vi "Main.vi"(7 "sweep rate, /min":dbl=0.2, 8 "sweep to:":dbl=-0.5, 9 "sweep":T6(radio)=enum."time_sweep") -> ()   [LabVIEW 2017] (continued)
                n3333 = property on="Figure_axis" class="Arr (strict)"("Value"=w4305) -> ()  [unwired: 2 in, 2 out]
                n3334 = property on="data_caption" class="Str"("Value"=w4307) -> ()  [unwired: 2 in, 2 out]
              }
              frame #32 {
                # "2182A 4 channel 1 measure (2182A_4_ch1)"
                n3335 = local read "2182A 4 ch1"() -> (w4324:bool)
                n3336 = property on="Figure_axis" class="Arr (strict)"() -> ("Value"=w4321:string[])  [unwired: 2 in, 2 out]
                n3337 = property on="data_caption" class="Str"() -> ("Value"=w4323:string)  [unwired: 2 in, 2 out]
                n3338 = case shown="True" w4324 {
                  tunnel: w4323 -> [w4326 w4332]
                  tunnel: [w4326 w4331] -> w4322
                  tunnel: w4321 -> [w4325 w4329]
                  tunnel: [w4325 w4327] -> w4320
                  frame False {
                    # "not measure 2182A 4 channel 1 (2182A_4_ch1)"
                  }
                  frame True {
                    w4328 = "2182A_4_ch1"
                    # "measure 2182A 4 channel 1 (2182A_4_ch1)"
                    n3339 = local read "2182A 4 addr"() -> (w4333:u8)
                    n3340 = Number To Decimal String(number=w4333) -> (decimal integer string=w4334:string)  [unwired: 1 in]
                    n3341 = GPIB Clear(3:w4334) -> ()  [unwired: 1 in, 2 out]
                    n3342 = Build Array (concatenate)(w4329, w4328) -> (w4327:string[])
                    n3343 = Concatenate Strings(w4332, w4328, "\t") -> (w4331:string)
                  }
                }
                n3344 = property on="Figure_axis" class="Arr (strict)"("Value"=w4320) -> ()  [unwired: 2 in, 2 out]
                n3345 = property on="data_caption" class="Str"("Value"=w4322) -> ()  [unwired: 2 in, 2 out]
              }
              frame #33 {
                # "2182A 4 channel 2 measure (2182A_4_ch2)"
                n3346 = local read "2182A 4 ch2"() -> (w4339:bool)
                n3347 = property on="Figure_axis" class="Arr (strict)"() -> ("Value"=w4336:string[])  [unwired: 2 in, 2 out]
                n3348 = property on="data_caption" class="Str"() -> ("Value"=w4338:string)  [unwired: 2 in, 2 out]
                n3349 = case shown="True" w4339 {
                  tunnel: w4338 -> [w4341 w4347]
                  tunnel: [w4341 w4346] -> w4337
                  tunnel: w4336 -> [w4340 w4344]
                  tunnel: [w4340 w4342] -> w4335
                  frame False {
                    # "not measure 2182A 4 channel 2 (2182A_4_ch2)"
                  }
                  frame True {
                    w4343 = "2182A_4_ch2"
                    # "measure 2182A 4 channel 2 (2182A_4_ch2)"
                    n3350 = local read "2182A 4 addr"() -> (w4348:u8)
                    n3351 = Number To Decimal String(number=w4348) -> (decimal integer string=w4349:string)  [unwired: 1 in]
                    n3352 = GPIB Clear(3:w4349) -> ()  [unwired: 1 in, 2 out]
                    n3353 = Build Array (concatenate)(w4344, w4343) -> (w4342:string[])
                    n3354 = Concatenate Strings(w4347, w4343, "\t") -> (w4346:string)
                  }
                }
                n3355 = property on="Figure_axis" class="Arr (strict)"("Value"=w4335) -> ()  [unwired: 2 in, 2 out]
                n3356 = property on="data_caption" class="Str"("Value"=w4337) -> ()  [unwired: 2 in, 2 out]
              }
              frame #34 {
                # "2636A smua measure voltage (2636A_smua_v)"
                n3357 = local read "2636A smua meas v"() -> (w4354:bool)
                n3358 = property on="Figure_axis" class="Arr (strict)"() -> ("Value"=w4351:string[])  [unwired: 2 in, 2 out]
                n3359 = property on="data_caption" class="Str"() -> ("Value"=w4353:string)  [unwired: 2 in, 2 out]
                n3360 = case shown="True" w4354 {
                  tunnel: w4353 -> [w4356 w4367]
                  tunnel: [w4356 w4366] -> w4352
                  tunnel: w4351 -> [w4355 w4364]
                  tunnel: [w4355 w4362] -> w4350
                  frame False {
                    # "not measure voltage on 2636A smua (2636A_smua_v)"
                  }
                  frame True {
                    w4363 = "2636A_smua_v"
                    # "measure voltage on 2636A smua (2636A_smua_v)"
                    n3361 = local read "2336A addr"() -> (w4358:refnum<visa-resource-name>)
                    n3362 = VISA Open(VISA resource name=w4358) -> (VISA resource name=w4357:refnum<visa-resource-name>, error out=w4359:errorcluster)  [unwired: 4 in]
                    n3363 = VISA Clear(VISA resource name=w4357, error in (no error)=w4359) -> (VISA resource name out=w4361:refnum<visa-resource-name>)  [unwired: 1 out]
                    n3364 = property class="Instr"(reference=w4361, "General Settings:Timeout Value"=u32 10000) -> ()  [unwired: 1 in, 2 out]
                    n3365 = Build Array (concatenate)(w4364, w4363) -> (w4362:string[])
                    n3366 = Concatenate Strings(w4367, w4363, "\t") -> (w4366:string)
                  }
                }
                n3367 = property on="Figure_axis" class="Arr (strict)"("Value"=w4350) -> ()  [unwired: 2 in, 2 out]
                n3368 = property on="data_caption" class="Str"("Value"=w4352) -> ()  [unwired: 2 in, 2 out]
              }
              frame #35 {
                # "2636A smua measure current (2636A_smua_i)"
                n3369 = local read "2636A smua meas i"() -> (w4372:bool)
                n3370 = property on="Figure_axis" class="Arr (strict)"() -> ("Value"=w4369:string[])  [unwired: 2 in, 2 out]
                n3371 = property on="data_caption" class="Str"() -> ("Value"=w4371:string)  [unwired: 2 in, 2 out]
                n3372 = case shown="True" w4372 {
                  tunnel: w4371 -> [w4374 w4385]
                  tunnel: [w4374 w4384] -> w4370
                  tunnel: w4369 -> [w4373 w4382]
                  tunnel: [w4373 w4380] -> w4368
                  frame False {
                    # "not measure current on 2636A smua (2636A_smua_i)"
                  }
                  frame True {
                    w4381 = "2636A_smua_i"
                    # "measure current on 2636A smua (2636A_smua_i)"
                    n3373 = local read "2336A addr"() -> (w4377:refnum<visa-resource-name>)
                    n3374 = VISA Open(VISA resource name=w4377) -> (VISA resource name=w4376:refnum<visa-resource-name>, error out=w4375:errorcluster)  [unwired: 4 in]
                    n3375 = VISA Clear(VISA resource name=w4376, error in (no error)=w4375) -> (VISA resource name out=w4378:refnum<visa-resource-name>)  [unwired: 1 out]
                    n3376 = Build Array (concatenate)(w4382, w4381) -> (w4380:string[])
                    n3377 = property class="Instr"(reference=w4378, "General Settings:Timeout Value"=u32 10000) -> ()  [unwired: 1 in, 2 out]
                    n3378 = Concatenate Strings(w4385, w4381, "\t") -> (w4384:string)
                  }
                }
                n3379 = property on="Figure_axis" class="Arr (strict)"("Value"=w4368) -> ()  [unwired: 2 in, 2 out]
                n3380 = property on="data_caption" class="Str"("Value"=w4370) -> ()  [unwired: 2 in, 2 out]
              }
              frame #36 {
                # "2636A smub measure voltage (2636A_smub_v)"
                n3381 = local read "2636A smub meas v"() -> (w4390:bool)
                n3382 = property on="Figure_axis" class="Arr (strict)"() -> ("Value"=w4387:string[])  [unwired: 2 in, 2 out]
                n3383 = property on="data_caption" class="Str"() -> ("Value"=w4389:string)  [unwired: 2 in, 2 out]
                n3384 = case shown="True" w4390 {
                  tunnel: w4389 -> [w4392 w4403]
                  tunnel: [w4392 w4402] -> w4388
                  tunnel: w4387 -> [w4391 w4400]
                  tunnel: [w4391 w4398] -> w4386
                  frame False {
                    # "not measure voltage on 2636A smub (2636A_smub_v)"
                  }
                  frame True {
                    w4399 = "2636A_smub_v"
                    # "measure voltage on 2636A smub (2636A_smub_v)"
                    n3385 = local read "2336A addr"() -> (w4394:refnum<visa-resource-name>)
                    n3386 = VISA Open(VISA resource name=w4394) -> (VISA resource name=w4393:refnum<visa-resource-name>, error out=w4395:errorcluster)  [unwired: 4 in]
                    n3387 = VISA Clear(VISA resource name=w4393, error in (no error)=w4395) -> (VISA resource name out=w4396:refnum<visa-resource-name>)  [unwired: 1 out]
                    n3388 = Build Array (concatenate)(w4400, w4399) -> (w4398:string[])
                    n3389 = property class="Instr"(reference=w4396, "General Settings:Timeout Value"=u32 10000) -> ()  [unwired: 1 in, 2 out]
                    n3390 = Concatenate Strings(w4403, w4399, "\t") -> (w4402:string)
                  }
                }
                n3391 = property on="Figure_axis" class="Arr (strict)"("Value"=w4386) -> ()  [unwired: 2 in, 2 out]
                n3392 = property on="data_caption" class="Str"("Value"=w4388) -> ()  [unwired: 2 in, 2 out]
              }
              frame #37 {
                # "2636A smub measure current (2636A_smub_i)"
                n3393 = local read "2636A smub meas i"() -> (w4408:bool)
                n3394 = property on="Figure_axis" class="Arr (strict)"() -> ("Value"=w4405:string[])  [unwired: 2 in, 2 out]
                n3395 = property on="data_caption" class="Str"() -> ("Value"=w4407:string)  [unwired: 2 in, 2 out]
                n3396 = case shown="True" w4408 {
                  tunnel: w4407 -> [w4410 w4421]
                  tunnel: [w4410 w4420] -> w4406
                  tunnel: w4405 -> [w4409 w4418]
                  tunnel: [w4409 w4416] -> w4404
                  frame False {
                    # "not measure current on 2636A smub (2636A_smub_i)"
                  }
                  frame True {
                    w4417 = "2636A_smub_i"
                    # "measure current on 2636A smub (2636A_smub_i)"
                    n3397 = local read "2336A addr"() -> (w4411:refnum<visa-resource-name>)
                    n3398 = VISA Open(VISA resource name=w4411) -> (VISA resource name=w4412:refnum<visa-resource-name>, error out=w4413:errorcluster)  [unwired: 4 in]
                    n3399 = VISA Clear(VISA resource name=w4412, error in (no error)=w4413) -> (VISA resource name out=w4414:refnum<visa-resource-name>)  [unwired: 1 out]
                    n3400 = Build Array (concatenate)(w4418, w4417) -> (w4416:string[])
                    n3401 = property class="Instr"(reference=w4414, "General Settings:Timeout Value"=u32 10000) -> ()  [unwired: 1 in, 2 out]
                    n3402 = Concatenate Strings(w4421, w4417, "\t") -> (w4420:string)
                  }
                }
                n3403 = property on="Figure_axis" class="Arr (strict)"("Value"=w4404) -> ()  [unwired: 2 in, 2 out]
                n3404 = property on="data_caption" class="Str"("Value"=w4406) -> ()  [unwired: 2 in, 2 out]
              }
              frame #38 {
                # "measure time"
                n3405 = local read "measure time"() -> (w4426:bool)
                n3406 = property on="Figure_axis" class="Arr (strict)"() -> ("Value"=w4423:string[])  [unwired: 2 in, 2 out]
                n3407 = property on="data_caption" class="Str"() -> ("Value"=w4425:string)  [unwired: 2 in, 2 out]
                n3408 = case shown="True" w4426 {
                  tunnel: w4425 -> [w4428 w4434]
                  tunnel: [w4428 w4433] -> w4424
                  tunnel: w4423 -> [w4427 w4431]
                  tunnel: [w4427 w4429] -> w4422
                  frame False {
                    # "not measuring time"
                  }
                  frame True {
                    w4430 = "time"
                    # "measuring time"
                    n3409 = Build Array (concatenate)(w4431, w4430) -> (w4429:string[])
                    n3410 = Concatenate Strings(w4434, w4430, "\t") -> (w4433:string)
                  }
                }
                n3411 = property on="Figure_axis" class="Arr (strict)"("Value"=w4422) -> ()  [unwired: 2 in, 2 out]
                n3412 = property on="data_caption" class="Str"("Value"=w4424) -> ()  [unwired: 2 in, 2 out]
              }
              frame #39 {
                # "Measure magnetic field on IPS120-0"
                n3413 = local read "iPS_MagnetField"() -> (w4439:bool)
                n3414 = property on="Figure_axis" class="Arr (strict)"() -> ("Value"=w4436:string[])  [unwired: 2 in, 2 out]
                n3415 = property on="data_caption" class="Str"() -> ("Value"=w4438:string)  [unwired: 2 in, 2 out]
                n3416 = case shown="True" w4439 {
                  tunnel: w4438 -> [w4441 w4447]
                  tunnel: [w4441 w4446] -> w4437
                  tunnel: w4436 -> [w4440 w4444]
                  tunnel: [w4440 w4442] -> w4435
                  frame False {
                    # "do not Measure magnetic field on IPS120-0"
                  }
                  frame True {
                    w4443 = "iPS_MagntField"
                    n3417 = Build Array (concatenate)(w4444, w4443) -> (w4442:string[])
                    n3418 = Concatenate Strings(w4447, w4443, "\t") -> (w4446:string)
                  }
                }
                n3419 = property on="Figure_axis" class="Arr (strict)"("Value"=w4435) -> ()  [unwired: 2 in, 2 out]
                n3420 = property on="data_caption" class="Str"("Value"=w4437) -> ()  [unwired: 2 in, 2 out]
              }
              frame #40 {
                # "Measure Magnet_T on iPS"
                n3421 = property on="Magnet_T" class="Bool (strict)"() -> ("Value"=w4448:bool)  [unwired: 2 in, 2 out]
                n3422 = property on="Figure_axis" class="Arr (strict)"() -> ("Value"=w4450:string[])  [unwired: 2 in, 2 out]
                n3423 = property on="data_caption" class="Str"() -> ("Value"=w4452:string)  [unwired: 2 in, 2 out]
                n3424 = case shown="True" w4448 {
                  tunnel: w4452 -> [w4454 w4460]
                  tunnel: [w4454 w4459] -> w4451
                  tunnel: w4450 -> [w4453 w4457]
                  tunnel: [w4453 w4455] -> w4449
                  frame False {
                    # "do not Measure magnetic field on IPS120-0"
                  }
                  frame True {
                    w4456 = "iPS_Magnet_T"
                    n3425 = Build Array (concatenate)(w4457, w4456) -> (w4455:string[])
                    n3426 = Concatenate Strings(w4460, w4456, "\t") -> (w4459:string)
                  }
                }
                n3427 = property on="Figure_axis" class="Arr (strict)"("Value"=w4449) -> ()  [unwired: 2 in, 2 out]
                n3428 = property on="data_caption" class="Str"("Value"=w4451) -> ()  [unwired: 2 in, 2 out]
              }
              frame #41 {
                # "Measure SH_T on iPS"
                n3429 = property on="SH_T" class="Bool (strict)"() -> ("Value"=w4461:bool)  [unwired: 2 in, 2 out]
                n3430 = property on="Figure_axis" class="Arr (strict)"() -> ("Value"=w4463:string[])  [unwired: 2 in, 2 out]
                n3431 = property on="data_caption" class="Str"() -> ("Value"=w4465:string)  [unwired: 2 in, 2 out]
                n3432 = case shown="False" w4461 {
                  tunnel: w4465 -> [w4467 w4473]
                  tunnel: [w4467 w4472] -> w4464
                  tunnel: w4463 -> [w4466 w4470]
                  tunnel: [w4466 w4468] -> w4462
                  frame False {
                    # "do not Measure magnetic field on IPS120-0"
                  }
                  frame True {
                    w4469 = "iPS_SH_T"
                    n3433 = Build Array (concatenate)(w4470, w4469) -> (w4468:string[])
                    n3434 = Concatenate Strings(w4473, w4469, "\t") -> (w4472:string)
                  }
                }
                n3435 = property on="Figure_axis" class="Arr (strict)"("Value"=w4462) -> ()  [unwired: 2 in, 2 out]
                n3436 = property on="data_caption" class="Str"("Value"=w4464) -> ()  [unwired: 2 in, 2 out]
              }
              frame #42 {
                # "iTC sample Temp"
                n3437 = property on="iTC_Sample_T" class="Bool (strict)"() -> ("Value"=w4474:bool)  [unwired: 2 in, 2 out]
                n3438 = property on="Figure_axis" class="Arr (strict)"() -> ("Value"=w4476:string[])  [unwired: 2 in, 2 out]
                n3439 = property on="data_caption" class="Str"() -> ("Value"=w4478:string)  [unwired: 2 in, 2 out]
                n3440 = case shown="True" w4474 {
                  tunnel: w4478 -> [w4480 w4486]
                  tunnel: [w4480 w4485] -> w4477
                  tunnel: w4476 -> [w4479 w4483]
                  tunnel: [w4479 w4481] -> w4475
                  frame False {
                    # "not measure 2461 voltage (2461_meas_v)"
                  }
                  frame True {
                    w4482 = "iTC_Sample_T"
                    n3441 = Build Array (concatenate)(w4483, w4482) -> (w4481:string[])
                    n3442 = Concatenate Strings(w4486, w4482, "\t") -> (w4485:string)
                  }
                }
                n3443 = property on="Figure_axis" class="Arr (strict)"("Value"=w4475) -> ()  [unwired: 2 in, 2 out]
                n3444 = property on="data_caption" class="Str"("Value"=w4477) -> ()  [unwired: 2 in, 2 out]
              }
              frame #43 {
                # "iTC sample Temp"
                n3445 = property on="VTI_T" class="Bool (strict)"() -> ("Value"=w4487:bool)  [unwired: 2 in, 2 out]
                n3446 = property on="Figure_axis" class="Arr (strict)"() -> ("Value"=w4489:string[])  [unwired: 2 in, 2 out]
                n3447 = property on="data_caption" class="Str"() -> ("Value"=w4491:string)  [unwired: 2 in, 2 out]
                n3448 = case shown="True" w4487 {
                  tunnel: w4491 -> [w4493 w4499]
                  tunnel: [w4493 w4498] -> w4490
                  tunnel: w4489 -> [w4492 w4496]
                  tunnel: [w4492 w4494] -> w4488
                  frame False {
                    # "not measure 2461 voltage (2461_meas_v)"
                  }
                  frame True {
                    w4495 = "iTC_VTI_T"
                    n3449 = Build Array (concatenate)(w4496, w4495) -> (w4494:string[])
                    n3450 = Concatenate Strings(w4499, w4495, "\t") -> (w4498:string)
                  }
                }
                n3451 = property on="Figure_axis" class="Arr (strict)"("Value"=w4488) -> ()  [unwired: 2 in, 2 out]
                n3452 = property on="data_caption" class="Str"("Value"=w4490) -> ()  [unwired: 2 in, 2 out]
              }
              frame #44 {
                # "iTC sample Temp"
                n3453 = property on="PT1_T" class="Bool (strict)"() -> ("Value"=w4500:bool)  [unwired: 2 in, 2 out]
                n3454 = property on="Figure_axis" class="Arr (strict)"() -> ("Value"=w4502:string[])  [unwired: 2 in, 2 out]
                n3455 = property on="data_caption" class="Str"() -> ("Value"=w4504:string)  [unwired: 2 in, 2 out]
                n3456 = case shown="True" w4500 {
                  tunnel: w4504 -> [w4506 w4512]
                  tunnel: [w4506 w4511] -> w4503
                  tunnel: w4502 -> [w4505 w4509]
                  tunnel: [w4505 w4507] -> w4501
                  frame False {
                    # "not measure 2461 voltage (2461_meas_v)"
                  }
                  frame True {
                    w4508 = "iTC_PT1_T"
                    n3457 = Build Array (concatenate)(w4509, w4508) -> (w4507:string[])
                    n3458 = Concatenate Strings(w4512, w4508, "\t") -> (w4511:string)
                  }
                }
                n3459 = property on="Figure_axis" class="Arr (strict)"("Value"=w4501) -> ()  [unwired: 2 in, 2 out]
                n3460 = property on="data_caption" class="Str"("Value"=w4503) -> ()  [unwired: 2 in, 2 out]
              }
              frame #45 {
                # "iTC sample Temp"
                n3461 = property on="PT2_T" class="Bool (strict)"() -> ("Value"=w4513:bool)  [unwired: 2 in, 2 out]
                n3462 = property on="Figure_axis" class="Arr (strict)"() -> ("Value"=w4515:string[])  [unwired: 2 in, 2 out]
                n3463 = property on="data_caption" class="Str"() -> ("Value"=w4517:string)  [unwired: 2 in, 2 out]
                n3464 = case shown="True" w4513 {
                  tunnel: w4517 -> [w4519 w4525]
                  tunnel: [w4519 w4524] -> w4516
                  tunnel: w4515 -> [w4518 w4522]
                  tunnel: [w4518 w4520] -> w4514
                  frame False {
                    # "not measure 2461 voltage (2461_meas_v)"
                  }
                  frame True {
                    w4521 = "iTC_PT2_T"
                    n3465 = Build Array (concatenate)(w4522, w4521) -> (w4520:string[])
                    n3466 = Concatenate Strings(w4525, w4521, "\t") -> (w4524:string)
                  }
                }
                n3467 = property on="Figure_axis" class="Arr (strict)"("Value"=w4514) -> ()  [unwired: 2 in, 2 out]
                n3468 = property on="data_caption" class="Str"("Value"=w4516) -> ()  [unwired: 2 in, 2 out]
              }
              frame #46 {
                # "iTC sample Temp"
                n3469 = property on="VTI_P" class="Bool (strict)"() -> ("Value"=w4526:bool)  [unwired: 2 in, 2 out]
                n3470 = property on="Figure_axis" class="Arr (strict)"() -> ("Value"=w4528:string[])  [unwired: 2 in, 2 out]
                n3471 = property on="data_caption" class="Str"() -> ("Value"=w4530:string)  [unwired: 2 in, 2 out]
                n3472 = case shown="True" w4526 {
                  tunnel: w4530 -> [w4532 w4538]
                  tunnel: [w4532 w4537] -> w4529
                  tunnel: w4528 -> [w4531 w4535]
                  tunnel: [w4531 w4533] -> w4527
                  frame False {
                    # "not measure 2461 voltage (2461_meas_v)"
                  }
                  frame True {
                    w4534 = "iTC_VTI_P"
                    n3473 = Build Array (concatenate)(w4535, w4534) -> (w4533:string[])
                    n3474 = Concatenate Strings(w4538, w4534, "\t") -> (w4537:string)
                  }
                }
                n3475 = property on="Figure_axis" class="Arr (strict)"("Value"=w4527) -> ()  [unwired: 2 in, 2 out]
                n3476 = property on="data_caption" class="Str"("Value"=w4529) -> ()  [unwired: 2 in, 2 out]
              }
              frame #47 {
                # "iTC sample Temp"
                n3477 = property on="2461_meas_v" class="Bool (strict)"() -> ("Value"=w4539:bool)  [unwired: 2 in, 2 out]
                n3478 = property on="Figure_axis" class="Arr (strict)"() -> ("Value"=w4541:string[])  [unwired: 2 in, 2 out]
                n3479 = property on="data_caption" class="Str"() -> ("Value"=w4543:string)  [unwired: 2 in, 2 out]
                n3480 = case shown="True" w4539 {
                  tunnel: w4543 -> [w4545 w4551]
                  tunnel: [w4545 w4550] -> w4542
                  tunnel: w4541 -> [w4544 w4548]
                  tunnel: [w4544 w4546] -> w4540
                  frame False {
                    # "not measure 2461 voltage (2461_meas_v)"
                  }
                  frame True {
                    w4547 = "2461_meas_v"
                    n3481 = Build Array (concatenate)(w4548, w4547) -> (w4546:string[])
                    n3482 = Concatenate Strings(w4551, w4547, "\t") -> (w4550:string)
                  }
                }
                n3483 = property on="Figure_axis" class="Arr (strict)"("Value"=w4540) -> ()  [unwired: 2 in, 2 out]
                n3484 = property on="data_caption" class="Str"("Value"=w4542) -> ()  [unwired: 2 in, 2 out]
              }
              frame #48 {
                # "iTC sample Temp"
                n3485 = property on="2461_meas_i" class="Bool (strict)"() -> ("Value"=w4552:bool)  [unwired: 2 in, 2 out]
                n3486 = property on="Figure_axis" class="Arr (strict)"() -> ("Value"=w4554:string[])  [unwired: 2 in, 2 out]
                n3487 = property on="data_caption" class="Str"() -> ("Value"=w4556:string)  [unwired: 2 in, 2 out]
                n3488 = case shown="True" w4552 {
                  tunnel: w4556 -> [w4558 w4564]
                  tunnel: [w4558 w4563] -> w4555
                  tunnel: w4554 -> [w4557 w4561]
                  tunnel: [w4557 w4559] -> w4553
                  frame False {
                    # "not measure 2461 voltage (2461_meas_v)"
                  }
                  frame True {
                    w4560 = "2461_meas_i"
                    n3489 = Build Array (concatenate)(w4561, w4560) -> (w4559:string[])
                    n3490 = Concatenate Strings(w4564, w4560, "\t") -> (w4563:string)
                  }
                }
                n3491 = property on="Figure_axis" class="Arr (strict)"("Value"=w4553) -> ()  [unwired: 2 in, 2 out]
                n3492 = property on="data_caption" class="Str"("Value"=w4555) -> ()  [unwired: 2 in, 2 out]
              }
              frame #49 {
                # "iTC sample Temp"
                n3493 = property on="Step Loop" class="Bool (strict)"() -> ("Value"=w4565:bool)  [unwired: 2 in, 2 out]
                n3494 = property on="Figure_axis" class="Arr (strict)"() -> ("Value"=w4567:string[])  [unwired: 2 in, 2 out]
                n3495 = property on="data_caption" class="Str"() -> ("Value"=w4569:string)  [unwired: 2 in, 2 out]
                n3496 = case shown="True" w4565 {
                  tunnel: w4569 -> [w4571 w4580]
                  tunnel: [w4571 w4579] -> w4568
                  tunnel: w4567 -> [w4570 w4577]
                  tunnel: [w4570 w4576] -> w4566
                  frame False {
                    # "not measure 2461 voltage (2461_meas_v)"
                  }
                  frame True {
                    n3497 = property on="step" class="RadioBtnsControl (strict)"() -> ("Value"=w4575:T8)  [unwired: 2 in, 2 out]
                    n3498 = case shown="\"iPS_step\"" w4575 {
                      tunnel: ["V2400_1" "V2400_2" "Va" "Vb" "time" "iTC" "iPS"] -> w4573
                      frame "V2400_1_Step", Default {
                      }
                      frame "V2400_2_step" {
                      }
                      frame "2636_smua_step" {
                      }
                      frame "2636_smub_step" {
                      }
                      frame "time_step" {
                      }
                      frame "iTC_step" {
                      }
                      frame "iPS_step" {
                      }
                    }
                    n3499 = Concatenate Strings(w4573, "_Step") -> (w4572:string)
                    n3500 = Build Array (concatenate)(w4577, w4572) -> (w4576:string[])
                    n3501 = Concatenate Strings(w4580, w4572, "\t") -> (w4579:string)
                  }
                }
                n3502 = property on="Figure_axis" class="Arr (strict)"("Value"=w4566) -> ()  [unwired: 2 in, 2 out]
                n3503 = property on="data_caption" class="Str"("Value"=w4568) -> ()  [unwired: 2 in, 2 out]
              }
              frame #50 {
                # "iTC sample Temp"
                n3504 = property on="HyperLoop" class="Bool (strict)"() -> ("Value"=w4588:bool)  [unwired: 2 in, 2 out]
                n3505 = property on="Figure_axis" class="Arr (strict)"() -> ("Value"=w4590:string[])  [unwired: 2 in, 2 out]
                n3506 = property on="data_caption" class="Str"() -> ("Value"=w4592:string)  [unwired: 2 in, 2 out]
                n3507 = case shown="True" w4588 {
                  tunnel: w4592 -> [w4594 w4603]
                  tunnel: [w4594 w4602] -> w4591
                  tunnel: w4590 -> [w4593 w4600]
                  tunnel: [w4593 w4599] -> w4589
                  frame False {
                    # "not measure 2461 voltage (2461_meas_v)"
                  }
                  frame True {
                    n3508 = property on="step_hyper" class="RadioBtnsControl (strict)"() -> ("Value"=w4598:T9)  [unwired: 2 in, 2 out]
                    n3509 = case shown="\"iPS_HyperLoop\"" w4598 {
                      tunnel: ["V2400_1" "V2400_2" "Va" "Vb" "time" "iTC" "iPS"] -> w4596
                      frame "2400_1_HyperLoop", Default {
                      }
                      frame "2400_2_HyperLoop" {
                      }
                      frame "2636_smua_HyperLoop" {
                      }
                      frame "2636_smub_HyperLoop" {
                      }
                      frame "time_HyperLoop" {
                      }
                      frame "iTC_HyperLoop" {
                      }
                      frame "iPS_HyperLoop" {
                      }
                    }
                    n3510 = Concatenate Strings(w4596, "_HyperLoop") -> (w4595:string)
                    n3511 = Build Array (concatenate)(w4600, w4595) -> (w4599:string[])
                    n3512 = Concatenate Strings(w4603, w4595, "\t") -> (w4602:string)
                  }
                }
                n3513 = property on="Figure_axis" class="Arr (strict)"("Value"=w4589) -> ()  [unwired: 2 in, 2 out]
                n3514 = property on="data_caption" class="Str"("Value"=w4591) -> ()  [unwired: 2 in, 2 out]
              }
              frame #51 {
                # "iTC sample Temp"
                n3515 = property on="SuperHyper" class="Bool (strict)"() -> ("Value"=w4611:bool)  [unwired: 2 in, 2 out]
                n3516 = property on="data_caption" class="Str"() -> ("Value"=w4615:string)  [unwired: 2 in, 2 out]
                n3517 = property on="Figure_axis" class="Arr (strict)"() -> ("Value"=w4613:string[])  [unwired: 2 in, 2 out]
                n3518 = case shown="True" w4611 {
                  tunnel: w4615 -> [w4617 w4626]
                  tunnel: [w4617 w4625] -> w4614
                  tunnel: w4613 -> [w4616 w4623]
                  tunnel: [w4616 w4622] -> w4612
                  frame False {
                    # "not measure 2461 voltage (2461_meas_v)"
                  }
                  frame True {
                    n3519 = property on="step_super" class="RadioBtnsControl (strict)"() -> ("Value"=w4618:T10)  [unwired: 2 in, 2 out]
                    n3520 = case shown="\"iTC_SuperHyper\"" w4618 {
                      tunnel: ["V2400_1" "V2400_2" "Va" "Vb" "time" "iTC" "iPS"] -> w4620
                      frame "2400_1_SuperHyper", Default {
                      }
                      frame "2400_2_SuperHyper" {
                      }
                      frame "2636_smua_SuperHyper" {
                      }
                      frame "2636_smub_SuperHyper" {
                      }
                      frame "time_SuperHyper" {
                      }
                      frame "iTC_SuperHyper" {
                      }
                      frame "iPS_SuperHyper" {
                      }
                    }
                    n3521 = Concatenate Strings(w4620, "_SuperHyper") -> (w4619:string)
                    n3522 = Build Array (concatenate)(w4623, w4619) -> (w4622:string[])
                    n3523 = Concatenate Strings(w4626, w4619, "\t") -> (w4625:string)
                  }
                }
                n3524 = property on="Figure_axis" class="Arr (strict)"("Value"=w4612) -> ()  [unwired: 2 in, 2 out]
                n3525 = property on="data_caption" class="Str"("Value"=w4614) -> ()  [unwired: 2 in, 2 out]
              }
            }
          }
          frame #2 {
            # "1 = 2400 1\n2 = 2400 2\n3 = 2400 3\n4 = 2636a smua\n5 = 2636a smub\n6 = do not sweep, just time\n7 = Teslatron_iPS_Field\n8 = Teslatron_iTC_Sample T"
            n3526 = property on="sweep" class="RadioBtnsControl (strict)"() -> ("Value"=w4634:T6)  [unwired: 2 in, 2 out]
            n3527 = case "reads current value from instrument which will be sweeping" shown="\"iPS\"" w4634 {
              tunnel: [w4636 w4646 w4655 w4664 w4668 0.0 ("Measuremet") w4674 w4694 w4697] -> w4635
              frame "2400_1", Default {
                # "reads the voltage on 2400 1"
                n3528 = local read "2400 1 addr"() -> (w4640:u8)
                n3529 = Number To Decimal String(number=w4640) -> (decimal integer string=w4641:string)  [unwired: 1 in]
                n3530 = GPIB Write(0:w4641, 1:":READ?") -> (6:w4637:errorcluster)  [unwired: 3 in, 1 out]
                n3531 = GPIB Read(0:w4641, 1:3200, 3:w4637) -> (5:w4643:string)  [unwired: 2 in, 2 out]
                n3532 = String Subset(string=w4643, length (rest)=13) -> (substring=w4644:string)  [unwired: 1 in]
                n3533 = Fract/Exp String To Number(string=w4644) -> (number=w4636:dbl)  [unwired: 3 in, 1 out]
              }
              frame "2400_2" {
                # "reads the current on 2400 2"
                n3534 = local read "2400 2 addr"() -> (w4650:u8)
                n3535 = Number To Decimal String(number=w4650) -> (decimal integer string=w4651:string)  [unwired: 1 in]
                n3536 = GPIB Write(0:w4651, 1:":READ?") -> (6:w4647:errorcluster)  [unwired: 3 in, 1 out]
                n3537 = GPIB Read(0:w4651, 1:3200, 3:w4647) -> (5:w4653:string)  [unwired: 2 in, 2 out]
                n3538 = String Subset(string=w4653, offset (0)=14, length (rest)=13) -> (substring=w4654:string)
                n3539 = Fract/Exp String To Number(string=w4654) -> (number=w4646:dbl)  [unwired: 3 in, 1 out]
              }
              frame "2400_3" {
                # "reads the voltage on 2400 3"
                n3540 = local read "2400 3 addr"() -> (w4659:u8)
                n3541 = Number To Decimal String(number=w4659) -> (decimal integer string=w4660:string)  [unwired: 1 in]
                n3542 = GPIB Write(0:w4660, 1:":READ?") -> (6:w4656:errorcluster)  [unwired: 3 in, 1 out]
                n3543 = GPIB Read(0:w4660, 1:3200, 3:w4656) -> (5:w4662:string)  [unwired: 2 in, 2 out]
                n3544 = String Subset(string=w4662, length (rest)=13) -> (substring=w4663:string)  [unwired: 1 in]
                n3545 = Fract/Exp String To Number(string=w4663) -> (number=w4655:dbl)  [unwired: 3 in, 1 out]
              }
              frame "2636a_smua" {
                # "reads the voltage on 2636a smua"
                n3546 = local read "2336A addr"() -> (w4667:refnum<visa-resource-name>)
                n3547 = call "SinglePointMeasurement.vi"("Measure"=Measure."Voltage", "Channel"=Channel."a", "VISA resource name 2"=w4667) -> ("Measuremet"=w4664:dbl)  [unwired: 3 in, 4 out]
              }
              frame "2636a_smub" {
                # "reads the voltage on 2636a smub"
                n3548 = local read "2336A addr"() -> (w4671:refnum<visa-resource-name>)
                n3549 = call "SinglePointMeasurement.vi"("Measure"=Measure."Voltage", "Channel"=Channel."b", "VISA resource name 2"=w4671) -> ("Measuremet"=w4668:dbl)  [unwired: 3 in, 4 out]
              }
              frame "time_sweep" {
              }
              frame "iPS" {
                n3550 = property on="Sweep B" class="Bool (strict)"() -> ("Value"=w4673:bool)  [unwired: 2 in, 2 out]
                n3551 = case shown="False" w4673 {
                  tunnel: [w4675 w4693] -> w4674
                  frame False {
                    n3552 = stacked-sequence {
                      tunnel: [_ _ w4682 _] -> w4675
                      frame #0 {
                        n3553 = local read "iPS_addr_sweep"() -> (w4678:refnum<visa-resource-name>)
                        n3554 = property on="sweep to:" class="DigNum (strict)"() -> ("Value"=w4676:dbl)  [unwired: 2 in, 2 out]
                        n3555 = call "iPSset.vi"("Target Field, T"=w4676, "iPSSetCtrl"=iPSsetCtrl."Set Target Field", "VISA resource name"=w4678) -> ()  [unwired: 5 in, 4 out]
                      }
                      frame #1 {
                        n3556 = local read "iPS_addr_sweep"() -> (w4681:refnum<visa-resource-name>)
                        n3557 = property on="sweep rate, /min" class="DigNum (strict)"() -> ("Value"=w4679:dbl)  [unwired: 2 in, 2 out]
                        n3558 = call "iPSset.vi"("Field Rate, T/min"=w4679, "iPSSetCtrl"=iPSsetCtrl."Set Target Field Rate", "VISA resource name"=w4681) -> ()  [unwired: 5 in, 4 out]
                      }
                      frame #2 {
                        n3559 = property on="iPS_addr_sweep" class="VISAName"() -> ("Value"=w4684:refnum<visa-resource-name>)  [unwired: 2 in, 2 out]
                        n3560 = call "iPSread.vi"("iPSreadCtrl"=iPSreadCtrl."OutputField", "VISA resource name"=w4684) -> ("number"=w4682:dbl)  [unwired: 6 in, 3 out]
                      }
                      frame #3 {
                        n3561 = property on="sweep to:" class="DigNum (strict)"() -> ("Value"=w4685:dbl)  [unwired: 2 in, 2 out]
                        n3562 = Not Equal To 0?(x=w4685) -> (x != 0?=w4688:bool)
                        n3563 = local read "iPS_addr_sweep"() -> (w4690:refnum<visa-resource-name>)
                        n3564 = Select(t=iPSsetCtrl."Go to Field" ("iPSSetCtrl"), s=w4688, f=iPSsetCtrl."Go to Field" ("iPSSetCtrl")) -> (s? t:f=w4686:T18)
                        n3565 = call "iPSset.vi"("iPSSetCtrl"=w4686, "VISA resource name"=w4690) -> ()  [unwired: 6 in, 4 out]
                      }
                    }
                  }
                  frame True {
                    # "Measure magnetic field on IPS120-0"
                    n3566 = property on="iPS_addr_sweep" class="VISAName"() -> ("Value"=w4692:refnum<visa-resource-name>)  [unwired: 2 in, 2 out]
                    n3567 = call "iPSread.vi"("iPSreadCtrl"=iPSreadCtrl."OutputField", "VISA resource name"=w4692) -> ("number"=w4693:dbl)  [unwired: 6 in, 3 out]
                  }
                }
              }
              frame "iTC" {
                n3568 = property on="iTC_addr_sweep" class="VISAName"() -> ("Value"=w4696:refnum<visa-resource-name>)  [unwired: 2 in, 2 out]
                n3569 = call "iTCread.vi"("VISA resource name"=w4696, "iTCreadCtrl"=iTCreadCtrl."Sample Temp") -> ("number"=w4694:dbl)  [unwired: 5 in, 3 out]
              }
              frame "2461" {
                n3570 = property on="2461_addr_sweep" class="VISAName"() -> ("Value"=w4698:refnum<visa-resource-name>)  [unwired: 2 in, 2 out]
                n3571 = call <instrlib>:"Get Source Level.vi"("VISA resource name"=w4698) -> ("Current Level Out"=w4697:dbl)  [unwired: 7 in, 3 out]
              }
            }
          }
          frame #3 {
            # "add \"formula\" string to the axis rings"
            n3572 = property on="Figure_axis" class="Arr (strict)"() -> ("Value"=w4701:string[])  [unwired: 2 in, 2 out]
            n3573 = Build Array (concatenate)(w4701, "formula") -> (w4699:string[])
            n3574 = property on="Figure_axis" class="Arr (strict)"("Value"=w4699) -> ()  [unwired: 2 in, 2 out]
          }
          frame #4 {
            # "passes array to ring"
            n3575 = property on="Figure_axis" class="Arr (strict)"() -> ("Value"=w4703:string[])  [unwired: 2 in, 2 out]
            n3576 = property on="Xaxis" class="Ring (strict)"("Strings []"=w4703) -> ()  [unwired: 2 in, 2 out]
            n3577 = property on="Yright" class="Ring (strict)"("Strings []"=w4703) -> ()  [unwired: 2 in, 2 out]
            n3578 = property on="Yaxis" class="Ring (strict)"("Strings []"=w4703) -> ()  [unwired: 2 in, 2 out]
            n3579 = property on="Stop Ramp" class="Bool"("DisabledEnum"=T12."Enabled" ("Disabled")) -> ()  [unwired: 2 in, 2 out]
          }
        }
        n3580 = call "timeInSeconds.vi"() -> ("Numeric"=w3757:dbl)  [unwired: 2 in, 1 out]
        n3581 = while {
          shift-right: [w4736] -> w3756
          shift-left: w3754 -> [w4735]
          tunnel: w3757 -> [w4733]
          shift-right: [w4727] -> _
          shift-left: w3753 -> [w4728]
          stop <- w4731 stop-if-true
          # "initial value"
          # "this loop stops when target value is reached"
          n3582 = stacked-sequence {
            tunnel: [_ _ w4825 _ _] -> w4730
            tunnel: [_ _ w4824 _ _] -> w4737
            tunnel: w4735 -> [_ _ w4818 _ _]
            tunnel: [w4810 _ _ _ _] -> w4734
            tunnel: w4733 -> [_ _ _ w4846 _]
            tunnel: [_ _ w4818 _ _] -> w4732
            tunnel: [_ _ _ _ w5505] -> w4726
            frame #0 {
              # "time is measured at the beginning\nand at the end of the cycle to\ncalculate delay time required to\nkeep set sweep rate"
              n3583 = flat-sequence {
                tunnel: [w4812] -> w4810
                frame #0 {
                  n3584 = property on="time delay, ms" class="DigNum (strict)"() -> ("Value"=w4811:dbl)  [unwired: 2 in, 2 out]
                  n3585 = Wait (ms)(milliseconds to wait=w4811) -> ()  [unwired: 1 out]
                }
                frame #1 {
                  n3586 = Tick Count (ms)() -> (millisecond timer value=w4812:u32)
                }
              }
            }
            frame #1 {
              w4813 = dbl[] []  # Empty array for data
              # "clear data array before each measurement cycle"
              n3587 = property on="data" class="Arr (strict)"("Value"=w4813) -> ()  [unwired: 2 in, 2 out]
            }
            frame #2 {
              # "add next sweep value to the data array"
              n3588 = property on="Sweep B" class="Bool (strict)"() -> ("Value"=w4815:bool)  [unwired: 2 in, 2 out]
              n3589 = local read "sweep"() -> (w4823:T6)
              n3590 = Not(x=w4815) -> (.not. x?=w4814:bool)
              n3591 = property on="data" class="Arr (strict)"() -> ("Value"=w4820:dbl[])  [unwired: 2 in, 2 out]
              n3592 = Equal?(x=w4823, y=T19."Radio Selection 7" ("sweep")) -> (x = y?=w4817:bool)
              n3593 = And(x=w4817, y=w4814) -> (x .and. y?=w4816:bool)
              n3594 = case shown="True" w4816 {
                tunnel: [w4827 w4844] -> w4825
                tunnel: [w4826 w4843] -> w4824
                tunnel: w4818 -> [_ w4839]
                tunnel: [w4826 w4839] -> w4819
                frame True {
                  # "sweeping magnetic field of Hulk"
                  n3595 = disable-structure shown="Disabled" {
                    frame Disabled {
                      n3596 = stacked-sequence {
                        tunnel: [_ w4835 _] -> _
                        tunnel: [_ _ w4837] -> _
                        frame #0 {
                          n3597 = local read "Hulk_SMS_addr"() -> (w4834:refnum<visa-resource-name>)
                          n3598 = VISA Clear(VISA resource name=w4834) -> ()  [unwired: 1 in, 2 out]
                        }
                        frame #1 {
                          # "acquires current output value"
                          n3599 = local read "Hulk_SMS_addr"() -> (w4836:refnum<visa-resource-name>)
                          n3600 = call "SMS_GET_OUTPUT.vi"("Hulk_SMS_addr"=w4836) -> ("Numeric"=w4835:dbl)  [unwired: 1 in, 2 out]
                        }
                        frame #2 {
                          # "checks, wheter ramp was finished"
                          n3601 = local read "Hulk_SMS_addr"() -> (w4838:refnum<visa-resource-name>)
                          n3602 = call "SMS_RAMP_STATUS.vi"("Hulk_SMS_addr"=w4838) -> ("selection"=w4837:bool)  [unwired: 1 in, 2 out]
                        }
                      }
                    }
                    frame Enabled {
                    }
                  }
                  n3603 = property on="iPS_addr_sweep" class="VISAName"() -> ("Value"=w4830:refnum<visa-resource-name>)  [unwired: 2 in, 2 out]
                  n3604 = property on="sweep to:" class="DigNum (strict)"() -> ("Value"=w4828:dbl)  [unwired: 2 in, 2 out]
                  n3605 = call "iPSread.vi"("iPSreadCtrl"=iPSreadCtrl."MagnetField", "VISA resource name"=w4830) -> ("number"=w4826:dbl)  [unwired: 6 in, 3 out]
                  n3606 = property on="Tolerance_Sweep" class="DigNum (strict)"() -> ("Value"=w4831:dbl)  [unwired: 2 in, 2 out]
                  n3607 = Subtract(x=w4826, y=w4828) -> (x-y=w4833:dbl)
                  n3608 = Absolute Value(x=w4833) -> (abs(x)=w4832:dbl)
                  n3609 = Less Or Equal?(x=w4832, y=w4831) -> (x <= y?=w4827:bool)
                }
                frame False {
                  # "calculate next value"
                  n3610 = property on="sweep to:" class="DigNum (strict)"() -> ("Value"=w4842:dbl)  [unwired: 2 in, 2 out]
                  n3611 = property on="sweep rate, /min" class="DigNum (strict)"() -> ("Value"=w4841:dbl)  [unwired: 2 in, 2 out]
                  n3612 = property on="time/point, sec" class="DigNum (strict)"() -> ("Value"=w4840:dbl)  [unwired: 2 in, 2 out]
                  n3613 = call "CalculateNextValue.vi"("Target a 2"=w4842, "Channel a source value"=w4839, "Ch a sweep rate units/min"=w4841, "time between points, sec"=w4840, "Source a"=Source."Voltage") -> ("Target a"=w4843:dbl, "Boolean"=w4844:bool)
                }
              }
              n3614 = Build Array (concatenate)(w4820, w4819) -> (w4821:dbl[])
              n3615 = property on="data" class="Arr (strict)"("Value"=w4821) -> ()  [unwired: 2 in, 2 out]
            }
            frame #3 {
              n3616 = stacked-sequence "measurement sequence" {
                tunnel: w4846 -> [_ _ _ _ _ _ _ _ _ _ _ _ _ _ _ _ _ _ _ _ _ _ _ _ _ _ _ _ _ _ _ _ _ _ _ _ _ _ w5384 _ _ _ _ _ _ _ _ _ _ _ _ _]
                frame #0 {
                  # "check if in-phase\nsignal on lock-in 1 \nis to be measured"
                  n3617 = property on="data" class="Arr (strict)"() -> ("Value"=w4848:dbl[])  [unwired: 2 in, 2 out]
                  n3618 = local read "SR830 1 ip"() -> (w4847:bool)
                  n3619 = case shown="True" w4847 {
                    tunnel: w4848 -> [w4850 w4859]
                    tunnel: [w4850 w4858] -> w4849
                    frame False {
                      # "we are not measuring in phase signal on lock-in 1 (SR830_1_ip)"
                    }
                    frame True {
                      # "we are  measuring lock-in 1, in phase (SR830_1_ip)"
                      n3620 = local read "SR830 1 addr"() -> (w4852:u8)
                      n3621 = Number To Decimal String(number=w4852) -> (decimal integer string=w4851:string)  [unwired: 1 in]
                      n3622 = GPIB Write(0:w4851, 1:"OUTR?1") -> (6:w4857:errorcluster)  [unwired: 3 in, 1 out]
                      n3623 = GPIB Read(0:w4851, 1:3200, 3:w4857) -> (5:w4855:string)  [unwired: 2 in, 2 out]
                      n3624 = Fract/Exp String To Number(string=w4855) -> (number=w4854:dbl)  [unwired: 3 in, 1 out]
                      n3625 = Build Array (concatenate)(w4859, w4854) -> (w4858:dbl[])
                    }
                  }
                  n3626 = property on="data" class="Arr (strict)"("Value"=w4849) -> ()  [unwired: 2 in, 2 out]
                }
                frame #1 {
                  # "check if out-of-phase\nsignal on lock-in 1 \nis to be measured"
                  n3627 = property on="data" class="Arr (strict)"() -> ("Value"=w4861:dbl[])  [unwired: 2 in, 2 out]
                  n3628 = local read "SR830 1 oop"() -> (w4860:bool)
                  n3629 = case shown="True" w4860 {
                    tunnel: w4861 -> [w4863 w4872]
                    tunnel: [w4863 w4871] -> w4862
                    frame False {
                      # "we are not measuring out of phase signal on lock-in 1 (SR830_1_oop)"
                    }
                    frame True {
                      # "we are  measuring lock-in 1, out of phase (SR830_1_oop)"
                      n3630 = local read "SR830 1 addr"() -> (w4865:u8)
                      n3631 = Number To Decimal String(number=w4865) -> (decimal integer string=w4864:string)  [unwired: 1 in]
                      n3632 = GPIB Write(0:w4864, 1:"OUTR?2") -> (6:w4870:errorcluster)  [unwired: 3 in, 1 out]
                      n3633 = GPIB Read(0:w4864, 1:3200, 3:w4870) -> (5:w4868:string)  [unwired: 2 in, 2 out]
                      n3634 = Fract/Exp String To Number(string=w4868) -> (number=w4867:dbl)  [unwired: 3 in, 1 out]
                      n3635 = Build Array (concatenate)(w4872, w4867) -> (w4871:dbl[])
                    }
                  }
                  n3636 = property on="data" class="Arr (strict)"("Value"=w4862) -> ()  [unwired: 2 in, 2 out]
                }
                frame #2 {
                  # "check if in-phase\nsignal on lock-in 2 \nis to be measured"
                  n3637 = property on="data" class="Arr (strict)"() -> ("Value"=w4874:dbl[])  [unwired: 2 in, 2 out]
                  n3638 = local read "SR830 2 ip"() -> (w4873:bool)
                  n3639 = case shown="True" w4873 {
                    tunnel: w4874 -> [w4876 w4885]
                    tunnel: [w4876 w4884] -> w4875
                    frame False {
                      # "we are not measuring in phase signal on lock-in 2 (SR830_2_ip)"
                    }
                    frame True {
                      # "we are  measuring lock-in 2, in phase (SR830_2_ip)"
                      n3640 = local read "SR830 2 addr"() -> (w4878:u8)
                      n3641 = Number To Decimal String(number=w4878) -> (decimal integer string=w4877:string)  [unwired: 1 in]
                      n3642 = GPIB Write(0:w4877, 1:"OUTP?1") -> (6:w4883:errorcluster)  [unwired: 3 in, 1 out]
                      n3643 = GPIB Read(0:w4877, 1:3200, 3:w4883) -> (5:w4881:string)  [unwired: 2 in, 2 out]
                      n3644 = Fract/Exp String To Number(string=w4881) -> (number=w4880:dbl)  [unwired: 3 in, 1 out]
                      n3645 = Build Array (concatenate)(w4885, w4880) -> (w4884:dbl[])
                    }
                  }
                  n3646 = property on="data" class="Arr (strict)"("Value"=w4875) -> ()  [unwired: 2 in, 2 out]
                }
                frame #3 {
                  # "check if out-of-phase\nsignal on lock-in 2 \nis to be measured"
                  n3647 = property on="data" class="Arr (strict)"() -> ("Value"=w4887:dbl[])  [unwired: 2 in, 2 out]
                  n3648 = local read "SR830 2 oop"() -> (w4886:bool)
                  n3649 = case shown="True" w4886 {
                    tunnel: w4887 -> [w4889 w4898]
                    tunnel: [w4889 w4897] -> w4888
                    frame False {
                      # "we are not measuring out of phase signal on lock-in 2 (SR830_2_oop)"
                    }
                    frame True {
                      # "we are  measuring lock-in 2, out of phase (SR830_2_oop)"
                      n3650 = local read "SR830 2 addr"() -> (w4891:u8)
                      n3651 = Number To Decimal String(number=w4891) -> (decimal integer string=w4890:string)  [unwired: 1 in]
                      n3652 = GPIB Write(0:w4890, 1:"OUTP?2") -> (6:w4896:errorcluster)  [unwired: 3 in, 1 out]
                      n3653 = GPIB Read(0:w4890, 1:3200, 3:w4896) -> (5:w4894:string)  [unwired: 2 in, 2 out]
                      n3654 = Fract/Exp String To Number(string=w4894) -> (number=w4893:dbl)  [unwired: 3 in, 1 out]
                      n3655 = Build Array (concatenate)(w4898, w4893) -> (w4897:dbl[])
                    }
                  }
                  n3656 = property on="data" class="Arr (strict)"("Value"=w4888) -> ()  [unwired: 2 in, 2 out]
                }
                frame #4 {
                  # "check if in-phase\nsignal on lock-in 3 \nis to be measured"
                  n3657 = property on="data" class="Arr (strict)"() -> ("Value"=w4900:dbl[])  [unwired: 2 in, 2 out]
                  n3658 = local read "SR830 3 ip"() -> (w4899:bool)
                  n3659 = case shown="True" w4899 {
                    tunnel: w4900 -> [w4902 w4911]
                    tunnel: [w4902 w4910] -> w4901
                    frame False {
                      # "we are not measuring in phase signal on lock-in 3 (SR830_3_ip)"
                    }
                    frame True {
                      # "we are  measuring lock-in 3, in phase (SR830_3_ip)"
                      n3660 = local read "SR830 3 addr"() -> (w4904:u8)
                      n3661 = Number To Decimal String(number=w4904) -> (decimal integer string=w4903:string)  [unwired: 1 in]
                      n3662 = GPIB Write(0:w4903, 1:"OUTP?1") -> (6:w4909:errorcluster)  [unwired: 3 in, 1 out]
                      n3663 = GPIB Read(0:w4903, 1:3200, 3:w4909) -> (5:w4907:string)  [unwired: 2 in, 2 out]
                      n3664 = Fract/Exp String To Number(string=w4907) -> (number=w4906:dbl)  [unwired: 3 in, 1 out]
                      n3665 = Build Array (concatenate)(w4911, w4906) -> (w4910:dbl[])
                    }
                  }
                  n3666 = property on="data" class="Arr (strict)"("Value"=w4901) -> ()  [unwired: 2 in, 2 out]
                }
                frame #5 {
                  # "check if out-of-phase\nsignal on lock-in 3 \nis to be measured"
                  n3667 = property on="data" class="Arr (strict)"() -> ("Value"=w4913:dbl[])  [unwired: 2 in, 2 out]
                  n3668 = local read "SR830 3 oop"() -> (w4912:bool)
                  n3669 = case shown="True" w4912 {
                    tunnel: w4913 -> [w4915 w4924]
                    tunnel: [w4915 w4923] -> w4914
                    frame False {
                      # "we are not measuring out of phase signal on lock-in 3 (SR830_3_oop)"
                    }
                    frame True {
                      # "we are  measuring lock-in 3, out of phase (SR830_3_oop)"
                      n3670 = local read "SR830 3 addr"() -> (w4917:u8)
                      n3671 = Number To Decimal String(number=w4917) -> (decimal integer string=w4916:string)  [unwired: 1 in]
                      n3672 = GPIB Write(0:w4916, 1:"OUTP?2") -> (6:w4922:errorcluster)  [unwired: 3 in, 1 out]
                      n3673 = GPIB Read(0:w4916, 1:3200, 3:w4922) -> (5:w4920:string)  [unwired: 2 in, 2 out]
                      n3674 = Fract/Exp String To Number(string=w4920) -> (number=w4919:dbl)  [unwired: 3 in, 1 out]
                      n3675 = Build Array (concatenate)(w4924, w4919) -> (w4923:dbl[])
                    }
                  }
                  n3676 = property on="data" class="Arr (strict)"("Value"=w4914) -> ()  [unwired: 2 in, 2 out]
                }
                frame #6 {
                  # "check if in-phase\nsignal on lock-in 4 \nis to be measured"
                  n3677 = property on="data" class="Arr (strict)"() -> ("Value"=w4926:dbl[])  [unwired: 2 in, 2 out]
                  n3678 = local read "SR830 4 ip"() -> (w4925:bool)
                  n3679 = case shown="True" w4925 {
                    tunnel: w4926 -> [w4928 w4937]
                    tunnel: [w4928 w4936] -> w4927
                    frame False {
                      # "we are not measuring in phase signal on lock-in 4 (SR830_4_ip)"
                    }
                    frame True {
                      # "we are  measuring lock-in 4, in phase (SR830_4_ip)"
                      n3680 = local read "SR830 4 addr"() -> (w4930:u8)
                      n3681 = Number To Decimal String(number=w4930) -> (decimal integer string=w4929:string)  [unwired: 1 in]
                      n3682 = GPIB Write(0:w4929, 1:"OUTP?1") -> (6:w4935:errorcluster)  [unwired: 3 in, 1 out]
                      n3683 = GPIB Read(0:w4929, 1:3200, 3:w4935) -> (5:w4933:string)  [unwired: 2 in, 2 out]
                      n3684 = Fract/Exp String To Number(string=w4933) -> (number=w4932:dbl)  [unwired: 3 in, 1 out]
                      n3685 = Build Array (concatenate)(w4937, w4932) -> (w4936:dbl[])
                    }
                  }
                  n3686 = property on="data" class="Arr (strict)"("Value"=w4927) -> ()  [unwired: 2 in, 2 out]
                }
                frame #7 {
                  # "check if out-of-phase\nsignal on lock-in 4 \nis to be measured"
                  n3687 = property on="data" class="Arr (strict)"() -> ("Value"=w4939:dbl[])  [unwired: 2 in, 2 out]
                  n3688 = local read "SR830 4 oop"() -> (w4938:bool)
                  n3689 = case shown="True" w4938 {
                    tunnel: w4939 -> [w4941 w4950]
                    tunnel: [w4941 w4949] -> w4940
                    frame False {
                      # "we are not measuring out of phase signal on lock-in 4 (SR830_4_oop)"
                    }
                    frame True {
                      # "we are  measuring lock-in 4, out of phase (SR830_4_oop)"
                      n3690 = local read "SR830 4 addr"() -> (w4943:u8)
                      n3691 = Number To Decimal String(number=w4943) -> (decimal integer string=w4942:string)  [unwired: 1 in]
                      n3692 = GPIB Write(0:w4942, 1:"OUTP?2") -> (6:w4948:errorcluster)  [unwired: 3 in, 1 out]
                      n3693 = GPIB Read(0:w4942, 1:3200, 3:w4948) -> (5:w4946:string)  [unwired: 2 in, 2 out]
                      n3694 = Fract/Exp String To Number(string=w4946) -> (number=w4945:dbl)  [unwired: 3 in, 1 out]
                      n3695 = Build Array (concatenate)(w4950, w4945) -> (w4949:dbl[])
                    }
                  }
                  n3696 = property on="data" class="Arr (strict)"("Value"=w4940) -> ()  [unwired: 2 in, 2 out]
                }
                frame #8 {
                  # "check if in-phase\nsignal on lock-in 5 \nis to be measured"
                  n3697 = property on="data" class="Arr (strict)"() -> ("Value"=w4952:dbl[])  [unwired: 2 in, 2 out]
                  n3698 = local read "SR830 5 ip"() -> (w4951:bool)
                  n3699 = case shown="True" w4951 {
                    tunnel: w4952 -> [w4954 w4963]
                    tunnel: [w4954 w4962] -> w4953
                    frame False {
                      # "we are not measuring in phase signal on lock-in 5 (SR830_5_ip)"
                    }
                    frame True {
                      # "we are  measuring lock-in 5 in phase (SR830_5_ip)"
                      n3700 = local read "SR830 5 addr"() -> (w4956:u8)
                      n3701 = Number To Decimal String(number=w4956) -> (decimal integer string=w4955:string)  [unwired: 1 in]
                      n3702 = GPIB Write(0:w4955, 1:"OUTP?1") -> (6:w4961:errorcluster)  [unwired: 3 in, 1 out]
                      n3703 = GPIB Read(0:w4955, 1:3200, 3:w4961) -> (5:w4959:string)  [unwired: 2 in, 2 out]
                      n3704 = Fract/Exp String To Number(string=w4959) -> (number=w4958:dbl)  [unwired: 3 in, 1 out]
                      n3705 = Build Array (concatenate)(w4963, w4958) -> (w4962:dbl[])
                    }
                  }
                  n3706 = property on="data" class="Arr (strict)"("Value"=w4953) -> ()  [unwired: 2 in, 2 out]
                }
                frame #9 {
                  # "check if out-of-phase\nsignal on lock-in 5 \nis to be measured"
                  n3707 = property on="data" class="Arr (strict)"() -> ("Value"=w4965:dbl[])  [unwired: 2 in, 2 out]
                  n3708 = local read "SR830 5 oop"() -> (w4964:bool)
                  n3709 = case shown="True" w4964 {
                    tunnel: w4965 -> [w4967 w4976]
                    tunnel: [w4967 w4975] -> w4966
                    frame False {
                      # "we are not measuring out of phase signal on lock-in 5 (SR830_5_oop)"
                    }
                    frame True {
                      # "we are  measuring lock-in 5 out of phase (SR830_5_oop)"
                      n3710 = local read "SR830 5 addr"() -> (w4969:u8)
